vi "global_motor.vi"() -> ()   [LabVIEW 2015]
panel:
  in  "_zero_point_steps_bypass":i32
  in  "_steps_per_turn":i32=200
  in  "_zero_point_steps":i32
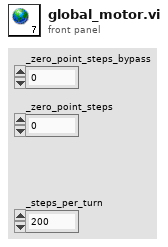
[diagram p1: front panel]
diagram:
